vi "CalculateGUIBinning.vi"(8 "error in (no error)":errorcluster, 11 "Photometrics_CH-250_Cam in":refnum<class "GenericCamera.lvclass">) -> (0 "error out":errorcluster, 3 "Photometrics_CH-250_Cam out":refnum<class "GenericCamera.lvclass">)   [LabVIEW 2013, in "GenericCamera.lvclass"]
uses:
  GenericCamera.lvclass
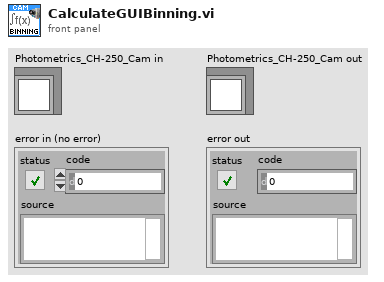
[diagram p1: front panel]
types:
  T1 = typedef "IMAQ Image.ctl" = refnum<image>
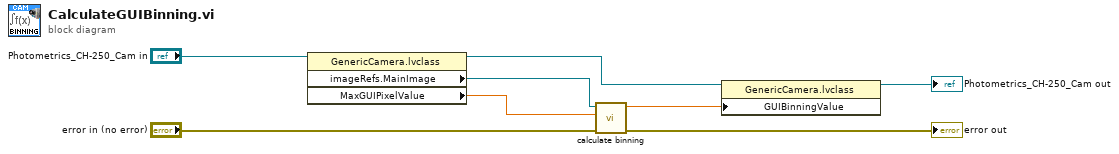
[diagram p0: block diagram]
diagram:
  n1 = property class="GenericCamera.lvclass"(reference="Photometrics_CH-250_Cam in") -> (reference out=w3:refnum<class "GenericCamera.lvclass">, "imageRefs.MainImage"=w5:T1, "MaxGUIPixelValue"=w4:dbl)  [unwired: 1 in, 1 out]
  n2 = call "calculate binning.vi"("error in (no error)"="error in (no error)", "MaxPixel"=w4, "ImageRefIn"=w5) -> ("error out"=→"error out":errorcluster, "BinningOut"=w2:dbl)  [unwired: 7 in]
  n3 = property class="GenericCamera.lvclass"(reference=w3, "GUIBinningValue"=w2) -> (reference out=→"Photometrics_CH-250_Cam out":refnum<class "GenericCamera.lvclass">)  [unwired: 1 in, 1 out]
